vi "testC.vi"(9 "Internal C":refnum<vi>, 11 "notifier out":refnum<notifier>) -> ()   [LabVIEW 2016]
panel:
  out "Numeric Control":i32
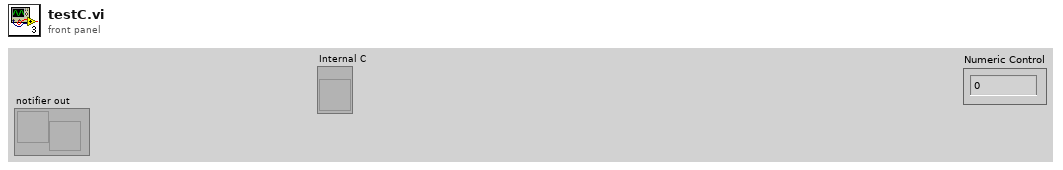
[diagram p1: front panel]
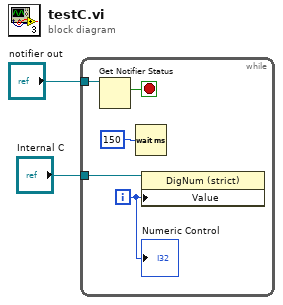
[diagram p0: block diagram]
diagram:
  n1 = while {
    tunnel: "notifier out" -> [w7]
    tunnel: "Internal C" -> [w3]
    i -> [w4]
    stop <- w6 stop-if-true
    n2 = Get Notifier Status(notifier=w7) -> (current notification=w6:bool)  [unwired: 1 in, 4 out]
    n3 = Wait (ms)(milliseconds to wait=u32 150) -> ()  [unwired: 1 out]
    n4 = property class="DigNum (strict)"(reference=w3, "Value"=w4) -> ()  [unwired: 1 in, 2 out]
    "Numeric Control" <- w4
  }
